vi "ActorDatabase-DeleteInstructions.vi"(7 "Payload From Actor":string, 8 "error in (no error)":errorcluster, 11 "Database-Actor in":refnum<class "PartCertDatabase-Actor.lvclass">) -> (0 "error out":errorcluster, 2 "New Payload":string, 3 "Database-Actor out":refnum<class "PartCertDatabase-Actor.lvclass">)   [LabVIEW 2013, in "PartCertDatabase-Actor.lvclass"]
uses:
  PartCertDatabase-Actor.lvclass
  PartCertDatabase-Actor.lvclass/PartCertDatabase-Actor.ctl
  Reuse Library/Database API/PartCertDatabase-API.lvclass
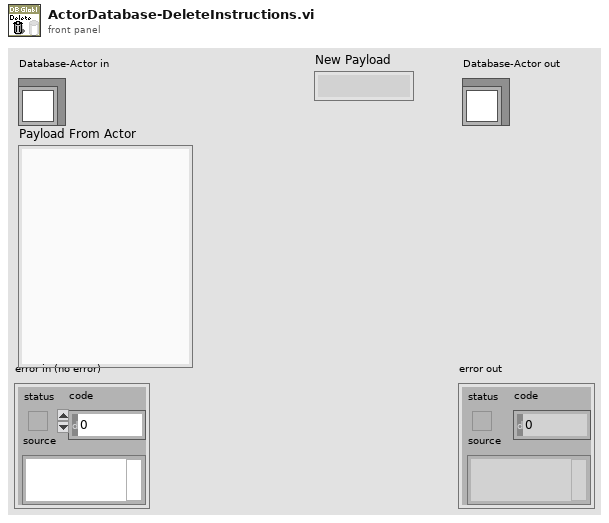
[diagram p1: front panel]
types:
  T1 = cluster{"Manufacturing-Part Number":string, "Array of Cluster Data":cluster{"Label Instructions":string, "Path for Picture Label":path, "Path for Picture Label 2":path, "Path for Picture Label 3":path, "Path for Picture Label 4":path, "Path for Picture Label 5":path, "Path for Picture Label 6":path, "Path for Picture Label 7":path, "Label Instructions 2":string, "Label Instructions 3":string}[], "Type of Insert":i32}
  T2 = cluster{"Table":string, "SQL Statement":string, "Update All":bool, "Payload":string, "Column Number":i32, "Datatype":i32, "Reply Command":string}
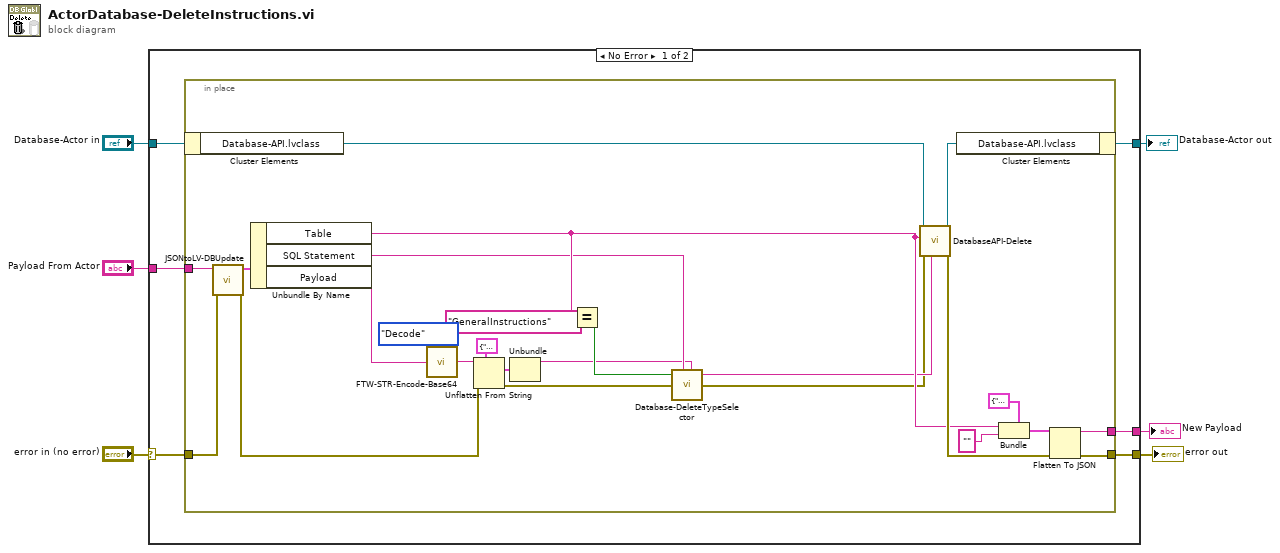
[diagram p0: block diagram]
diagram:
  n1 = case shown="No Error" "error in (no error)" {
    selector: "error in (no error)" -> [w10 w39]
    tunnel: [w8 w39] -> w5
    tunnel: [w11 w38] -> w3
    tunnel: "Database-Actor in" -> [w12 w38]
    tunnel: "Payload From Actor" -> [w9 _]
    tunnel: [w7 _] -> w1
    frame No Error {
      n2 = in-place {
        in-place-border: w10 -> [w37]
        in-place-border: w9 -> [w35]
        in-place-border: [w25] -> w8
        in-place-border: [w21] -> w7
        n3 = in-place-cluster #1(w12) -> ("Database-API.lvclass"=w34:refnum<class "PartCertDatabase-API.lvclass">)
        n4 = call "JSONtoLV-DBUpdate.vi"("error in"=w37, "Input JSON Object"=w35) -> ("error out"=w27:errorcluster, "value"=w36:T2)  [unwired: 8 in]
        n5 = Unbundle By Name(w36) -> ("Table"=w18:string, "SQL Statement"=w16:string, "Payload"=w31:string)
        n6 = call "FTW-STR-Encode-Base64.vi"("Input"=w31, "Direction"=enum16{"Encode", "Decode"}."Decode") -> ("Output"=w28:string)
        n7 = Unflatten From String(type=T1 {"Manufacturing-Part Number"="", "Array of Cluster Data"=[], "Type of Insert"=0} ("cluster"), binary string=w28, error in (no error)=w27) -> (value=w29:T1, error out=w14:errorcluster)  [unwired: 2 in, 1 out]
        n8 = Unbundle(w29) -> ("Manufacturing-Part Number"=w15:string)  [unwired: 2 out]
        n9 = Equal?(x=w18, y="GeneralInstructions") -> (x = y?=w19:bool)
        n10 = call "Database-DeleteTypeSelector.vi"("General Instruction"=w19, "SQL Statement"=w16, "error in (no error)"=w14, "Manufacturing-Part Number"=w15) -> ("SQL"=w17:string, "error out"=w13:errorcluster)  [unwired: 4 in]
        n11 = call "DatabaseAPI-Delete.vi"("Where Statement"=w17, "error in (no error)"=w13, "table"=w18, "Database-API in"=w34) -> ("error out"=w26:errorcluster, "Database-API out"=w33:refnum<class "PartCertDatabase-API.lvclass">)  [unwired: 6 in]
        n12 = in-place-cluster #1("Database-API.lvclass"=w33) -> (w11:refnum<class "PartCertDatabase-Actor.lvclass">)
        n13 = Bundle(cluster=cluster{"Table":string, "SQL Statement":string} {"Table"="", "SQL Statement"=""}, "Table"=w18, "SQL Statement"="") -> (w22:cluster{"Table":string, "SQL Statement":string})
        n14 = Flatten To JSON(anything=w22, error in (no error)=w26) -> (JSON string=w21:string, 11:w25:errorcluster)  [unwired: 1 in]
      }
    }
    frame Error {
    }
  }
  "error out" <- w5
  "Database-Actor out" <- w3
  "New Payload" <- w1
